vi "状态输出.vi"() -> (3 "采配水流程":T1(ring)=enum."结束")   [LabVIEW 2016, in "PLC.lvlib"]
uses:
  PLC.lvlib
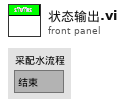
[diagram p1: front panel]
types:
  T1 = enum16{"空闲", "润洗", "采样", "沉淀", "配水", "反冲洗", "储水", "结束"}
  T2 = cluster{"R0":i16, "R1":i16, "R2":i16, "R3":i16, "R4":i16, "R5":i16, "R6":i16, "R7":i16, "R8":i16, "R9":i16, "R10":i16, "R11":i16, "R12":i16, "R13":i16, "R14":i16, "R15":i16, "R16":i16, "R17":i16, "R18":i16, "R19":i16, "R20":i16, "R21":i16, "R22":i16, "R23":i16, "R24":i16, "R25":i16, "R26":i16, "R27":i16, "R28":i16, "R29":i16, "R30":i16, "R31":i16, "R32":i16, "R33":i16, "R34":i16, "R35":i16, "R36":i16, "R37":i16, "R38":i16, "R39":i16, "R40":i16, "R41":i16, "R42":i16, "R43":i16, "R44":i16, "R45":i16, "R46":i16, "R47":i16, "R48":i16, "R49":i16, "R50":i16, "R51":i16, "R52":i16, "R53":i16, "R54":i16, "R55":i16, "R56":i16, "R57":i16, "R58":i16, "R59":i16, "R60":i16, "R61":i16, "R62":i16, "R63":i16, "R64":i16, "R65":i16, "R66":i16, "R67":i16, "R68":i16, "R69":i16, "R70":i16, "R71":i16, "R72":i16, "R73":i16, "R74":i16, "R75":i16, "R76":i16, "R77":i16, "R78":i16, "R79":i16}
  T3 = typedef "采配水类型.ctl" = enum16{"V1", "V2", "V3", "V4", "室内V1", "室内V2", "固定站V1", "固定站V2", "浮船V1", "浮船V2"}
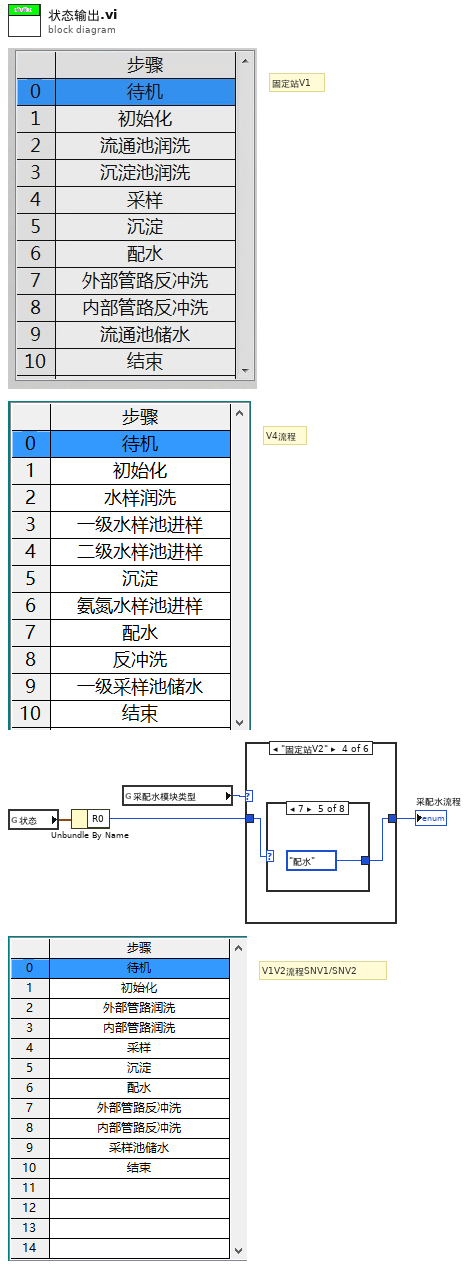
[diagram p0: block diagram]
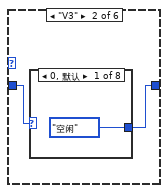
[diagram p3: hidden frame]
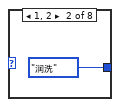
[diagram p4: hidden frame]
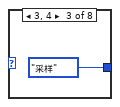
[diagram p5: hidden frame]
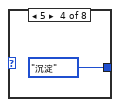
[diagram p6: hidden frame]
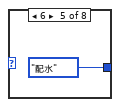
[diagram p7: hidden frame]
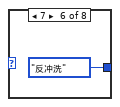
[diagram p8: hidden frame]
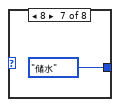
[diagram p9: hidden frame]
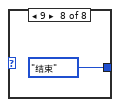
[diagram p10: hidden frame]
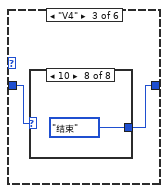
[diagram p11: hidden frame]
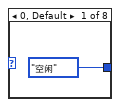
[diagram p12: hidden frame]
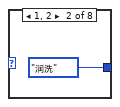
[diagram p13: hidden frame]
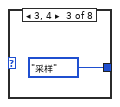
[diagram p14: hidden frame]
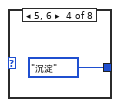
[diagram p15: hidden frame]
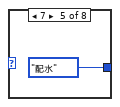
[diagram p16: hidden frame]
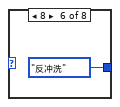
[diagram p17: hidden frame]
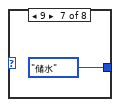
[diagram p18: hidden frame]
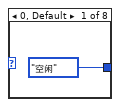
[diagram p19: hidden frame]
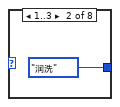
[diagram p20: hidden frame]
diagram:
  # "固定站V1"
  # "V1V2流程SNV1/SNV2"
  # "V4流程"
  n1 = global read "采配水全局变量.vi" "状态"() -> (w4:T2)
  n2 = Unbundle By Name(w4) -> ("R0"=w3:i16)
  n3 = global read "系统设置全局变量.vi" "采配水模块类型"() -> (w2:T3)
  n4 = case shown="\"固定站V2\"" w2 {
    tunnel: w3 -> [w5 w7 w17 w27 w37 w47]
    tunnel: [w5 w6 w16 w26 w36 w46] -> w1
    frame Default {
    }
    frame "V3" {
      n5 = case shown="0, 默认" w7 {
        tunnel: [T1."空闲" ("采配水流程") T1."润洗" ("采配水流程") T1."采样" ("采配水流程") T1."沉淀" ("采配水流程") T1."配水" ("采配水流程") T1."反冲洗" ("采配水流程") T1."储水" ("采配水流程") T1."结束" ("采配水流程")] -> w6
        frame 0, Default {
        }
        frame 1, 2 {
        }
        frame 3, 4 {
        }
        frame 5 {
        }
        frame 6 {
        }
        frame 7 {
        }
        frame 8 {
        }
        frame 9 {
        }
      }
    }
    frame "V4" {
      n6 = case shown="10" w17 {
        tunnel: [T1."空闲" ("采配水流程") T1."润洗" ("采配水流程") T1."采样" ("采配水流程") T1."沉淀" ("采配水流程") T1."配水" ("采配水流程") T1."反冲洗" ("采配水流程") T1."储水" ("采配水流程") T1."结束" ("采配水流程")] -> w16
        frame 0, Default {
        }
        frame 1, 2 {
        }
        frame 3, 4 {
        }
        frame 5, 6 {
        }
        frame 7 {
        }
        frame 8 {
        }
        frame 9 {
        }
        frame 10 {
        }
      }
    }
    frame "固定站V2" {
      n7 = case shown="7" w27 {
        tunnel: [T1."空闲" ("采配水流程") T1."润洗" ("采配水流程") T1."采样" ("采配水流程") T1."沉淀" ("采配水流程") T1."配水" ("采配水流程") T1."反冲洗" ("采配水流程") T1."储水" ("采配水流程") T1."结束" ("采配水流程")] -> w26
        frame 0, Default {
        }
        frame 1..3 {
        }
        frame 4 {
        }
        frame 5, 6 {
        }
        frame 7 {
        }
        frame 8, 9 {
        }
        frame 10 {
        }
        frame 11 {
        }
      }
    }
    frame "固定站V1" {
      n8 = case shown="10" w37 {
        tunnel: [T1."空闲" ("采配水流程") T1."润洗" ("采配水流程") T1."采样" ("采配水流程") T1."沉淀" ("采配水流程") T1."配水" ("采配水流程") T1."反冲洗" ("采配水流程") T1."储水" ("采配水流程") T1."结束" ("采配水流程")] -> w36
        frame 0, Default {
        }
        frame 1..3 {
        }
        frame 4 {
        }
        frame 5 {
        }
        frame 6 {
        }
        frame 7, 8 {
        }
        frame 9 {
        }
        frame 10 {
        }
      }
    }
    frame "V1", "V2", "室内V1", "室内V2" {
      n9 = case shown="10" w47 {
        tunnel: [T1."空闲" ("采配水流程") T1."润洗" ("采配水流程") T1."采样" ("采配水流程") T1."沉淀" ("采配水流程") T1."配水" ("采配水流程") T1."反冲洗" ("采配水流程") T1."储水" ("采配水流程") T1."结束" ("采配水流程")] -> w46
        frame 0, Default {
        }
        frame 1..3 {
        }
        frame 4 {
        }
        frame 5 {
        }
        frame 6 {
        }
        frame 7, 8 {
        }
        frame 9 {
        }
        frame 10 {
        }
      }
    }
  }
  "采配水流程" <- w1
